vi "Mappa AO PLC_3.vi"(10 "USCITE PLC":T1) -> (0 "Array DB REAL out":dbl[](array[numeric]), 1 "Array DB W out":dbl[](array[numeric]), 2 "Array M REAL out":dbl[](array[numeric]), 3 "Array M WORD out":dbl[](array[numeric]))   [LabVIEW 2019]
uses:
  Uscite PLC 3.ctl
  controls/statoAO_plc_3.ctl
  StatoDO_PLC_3.ctl
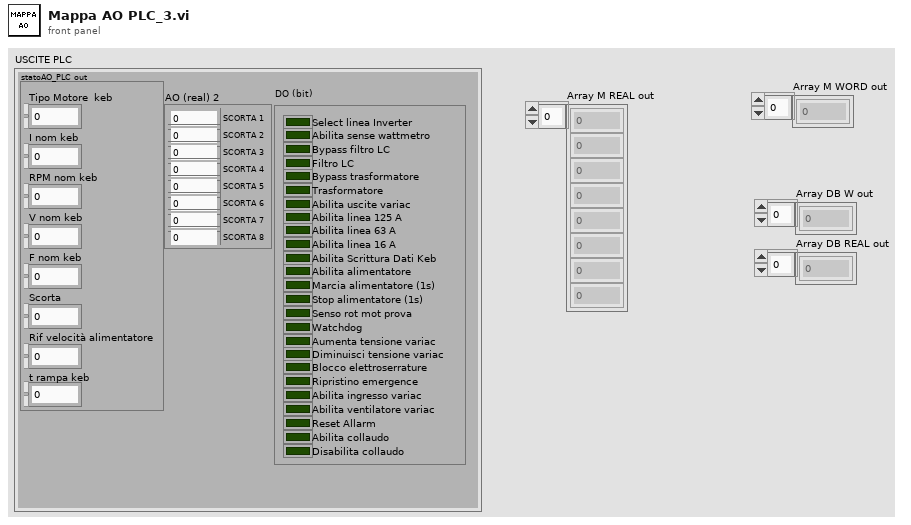
[diagram p1: front panel]
types:
  T1 = typedef "Uscite PLC 3.ctl" = cluster{"AO (real) 2":cluster{"SCORTA 1":dbl, "SCORTA 2":dbl, "SCORTA 3":dbl, "SCORTA 4":dbl, "SCORTA 5":dbl, "SCORTA 6":dbl, "SCORTA 7":dbl, "SCORTA 8":dbl}, "statoAO_PLC out":T2, "DO (bit)":T3}
  T2 = typedef "statoAO_plc_3.ctl" = cluster{"Rif velocità alimentatore":dbl, "Scorta":dbl, "Tipo Motore  keb":dbl, "I nom keb":dbl, "RPM nom keb":dbl, "V nom keb":dbl, "F nom keb":dbl, "t rampa keb":dbl}
  T3 = typedef "StatoDO_PLC_3.ctl" = cluster{"Select linea Inverter":bool, "Abilita sense wattmetro":bool, "Bypass filtro LC":bool, "Filtro LC":bool, "Bypass trasformatore":bool, "Trasformatore":bool, "Abilita uscite variac":bool, "Abilita linea 125 A":bool, "Abilita linea 63 A":bool, "Abilita linea 16 A":bool, "Abilita Scrittura Dati Keb":bool, "Abilita alimentatore":bool, "Marcia alimentatore (1s)":bool, "Stop alimentatore (1s)":bool, "Senso rot mot prova":bool, "Watchdog":bool, "Aumenta tensione variac":bool, "Diminuisci tensione variac ":bool, "Blocco elettroserrature":bool, "Ripristino emergence":bool, "Abilita ingresso variac":bool, "Abilita ventilatore variac":bool, "Reset Allarm":bool, "Scorta 1":bool, "Scorta 2":bool, "Scorta 3":bool, "Scorta 4":bool, "Scorta 5":bool, "Scorta 6":bool, "Scorta 7":bool, "Scorta 8":bool, "Scorta 9":bool, "Abilita collaudo":bool, "Disabilita collaudo ":bool, "Scorta 10":bool, "Scorta 11":bool, "Scorta 12":bool, "Scorta 13":bool, "Scorta 14":bool, "Scorta 15":bool}
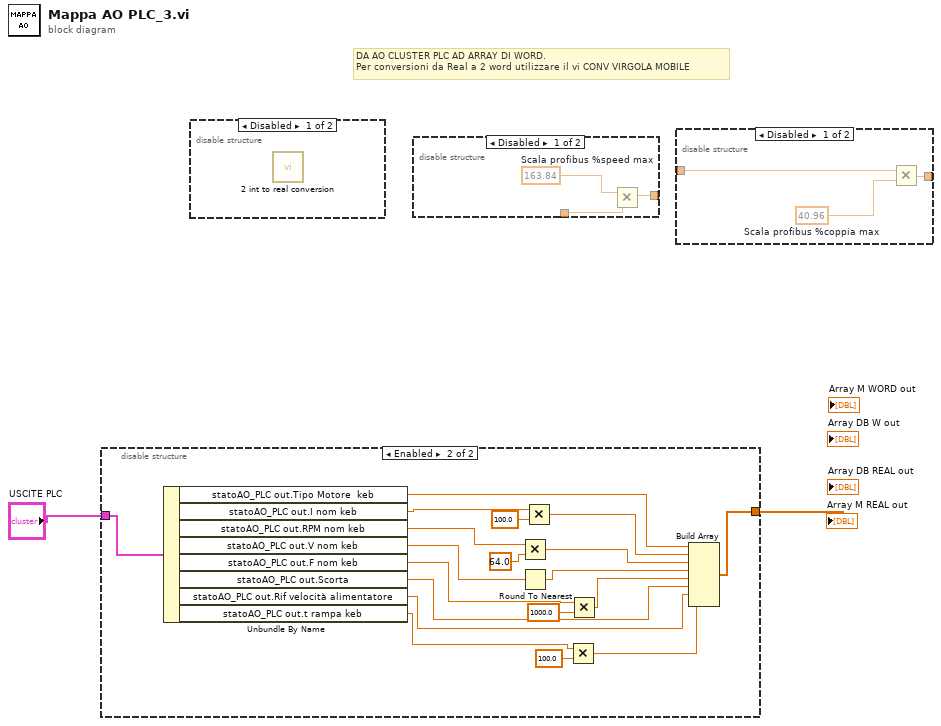
[diagram p0: block diagram]
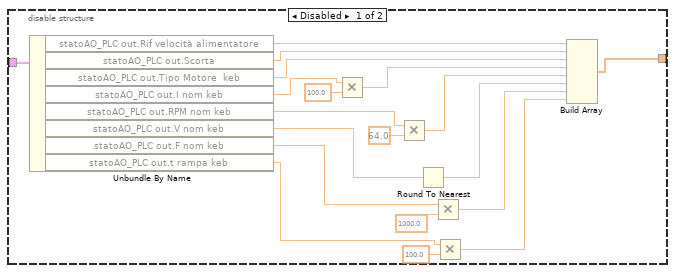
[diagram p2: hidden frame]
diagram:
  # "DA AO CLUSTER PLC AD ARRAY DI WORD.\nPer conversioni da Real a 2 word utilizzare il vi CONV VIRGOLA MOBILE"
  n1 = disable-structure shown="Enabled" {
    disable-tunnel: [w9 w22] -> w2
    disable-tunnel: "USCITE PLC" -> [w3 w23]
    frame Disabled {
      n2 = Unbundle By Name(w3) -> ("statoAO_PLC out.Rif velocità alimentatore"=w21:dbl, "statoAO_PLC out.Scorta"=w20:dbl, "statoAO_PLC out.Tipo Motore  keb"=w19:dbl, "statoAO_PLC out.I nom keb"=w17:dbl, "statoAO_PLC out.RPM nom keb"=w14:dbl, "statoAO_PLC out.V nom keb"=w8:dbl, "statoAO_PLC out.F nom keb"=w11:dbl, "statoAO_PLC out.t rampa keb"=w5:dbl)
      n3 = Multiply(x=w17, y=100.0) -> (x*y=w16:dbl)
      n4 = Multiply(x=w14, y=64.0) -> (x*y=w13:dbl)
      n5 = Round To Nearest(number=w8) -> (nearest integer value=w7:dbl)
      n6 = Multiply(x=w11, y=1000.0) -> (x*y=w10:dbl)
      n7 = Multiply(x=w5, y=100.0) -> (x*y=w4:dbl)
      n8 = Build Array(w21, w20, w19, w16, w13, w7, w10, w4) -> (w9:dbl[])
    }
    frame Enabled {
      n9 = Unbundle By Name(w23) -> ("statoAO_PLC out.Tipo Motore  keb"=w28:dbl, "statoAO_PLC out.I nom keb"=w29:dbl, "statoAO_PLC out.RPM nom keb"=w31:dbl, "statoAO_PLC out.V nom keb"=w33:dbl, "statoAO_PLC out.F nom keb"=w35:dbl, "statoAO_PLC out.Scorta"=w37:dbl, "statoAO_PLC out.Rif velocità alimentatore"=w38:dbl, "statoAO_PLC out.t rampa keb"=w39:dbl)
      n10 = Multiply(x=w31, y=64.0) -> (x*y=w32:dbl)
      n11 = Round To Nearest(number=w33) -> (nearest integer value=w34:dbl)
      n12 = Multiply(x=w29, y=100.0) -> (x*y=w30:dbl)
      n13 = Multiply(x=w39, y=100.0) -> (x*y=w40:dbl)
      n14 = Multiply(x=w35, y=1000.0) -> (x*y=w36:dbl)
      n15 = Build Array(w28, w30, w32, w34, w36, w37, w38, w40) -> (w22:dbl[])
    }
  }
  "Array M REAL out" <- w2
  n16 = disable-structure shown="Disabled" {
    frame Disabled {
      n17 = call "2 int to real conversion.vi"() -> ()  [unwired: 9 in, 3 out]
    }
    frame Enabled {
    }
  }
  n18 = disable-structure shown="Disabled" {
    disable-tunnel: _ -> [w43 _]
    disable-tunnel: [w42 _] -> _
    frame Disabled {
      w41 = 163.84  # Scala profibus %speed max
      n19 = Multiply(x=w41, y=w43) -> (x*y=w42:dbl)
    }
    frame Enabled {
    }
  }
  n20 = disable-structure shown="Disabled" {
    disable-tunnel: _ -> [w46 _]
    disable-tunnel: [w45 _] -> _
    frame Disabled {
      w44 = 40.96  # Scala profibus %coppia max
      n21 = Multiply(x=w46, y=w44) -> (x*y=w45:dbl)
    }
    frame Enabled {
    }
  }
